vi "testTwoClientsSendCmdAtSameTime.vi"(8 "error in":errorcluster) -> (0 "error out":errorcluster)   [LabVIEW 2018]
uses:
  src/FactoryTcpServer/FactoryTcpServer.lvclass
  <vilib>/addons/_JKI Toolkits/Caraya/classes/Assert/Assert Equal Value_Variant.vi
  src/TcpServer/TcpServer.lvclass
  <vilib>/addons/_JKI Toolkits/Caraya/classes/Test/Test.lvclass
  <vilib>/addons/_JKI Toolkits/Caraya/classes/Assert/Assert.lvclass
panel:
  out "Run Server B error":errorcluster
  out "Run Server A error":errorcluster
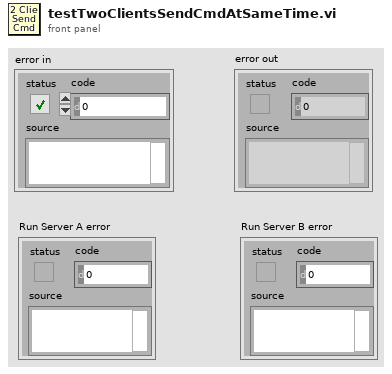
[diagram p1: front panel]
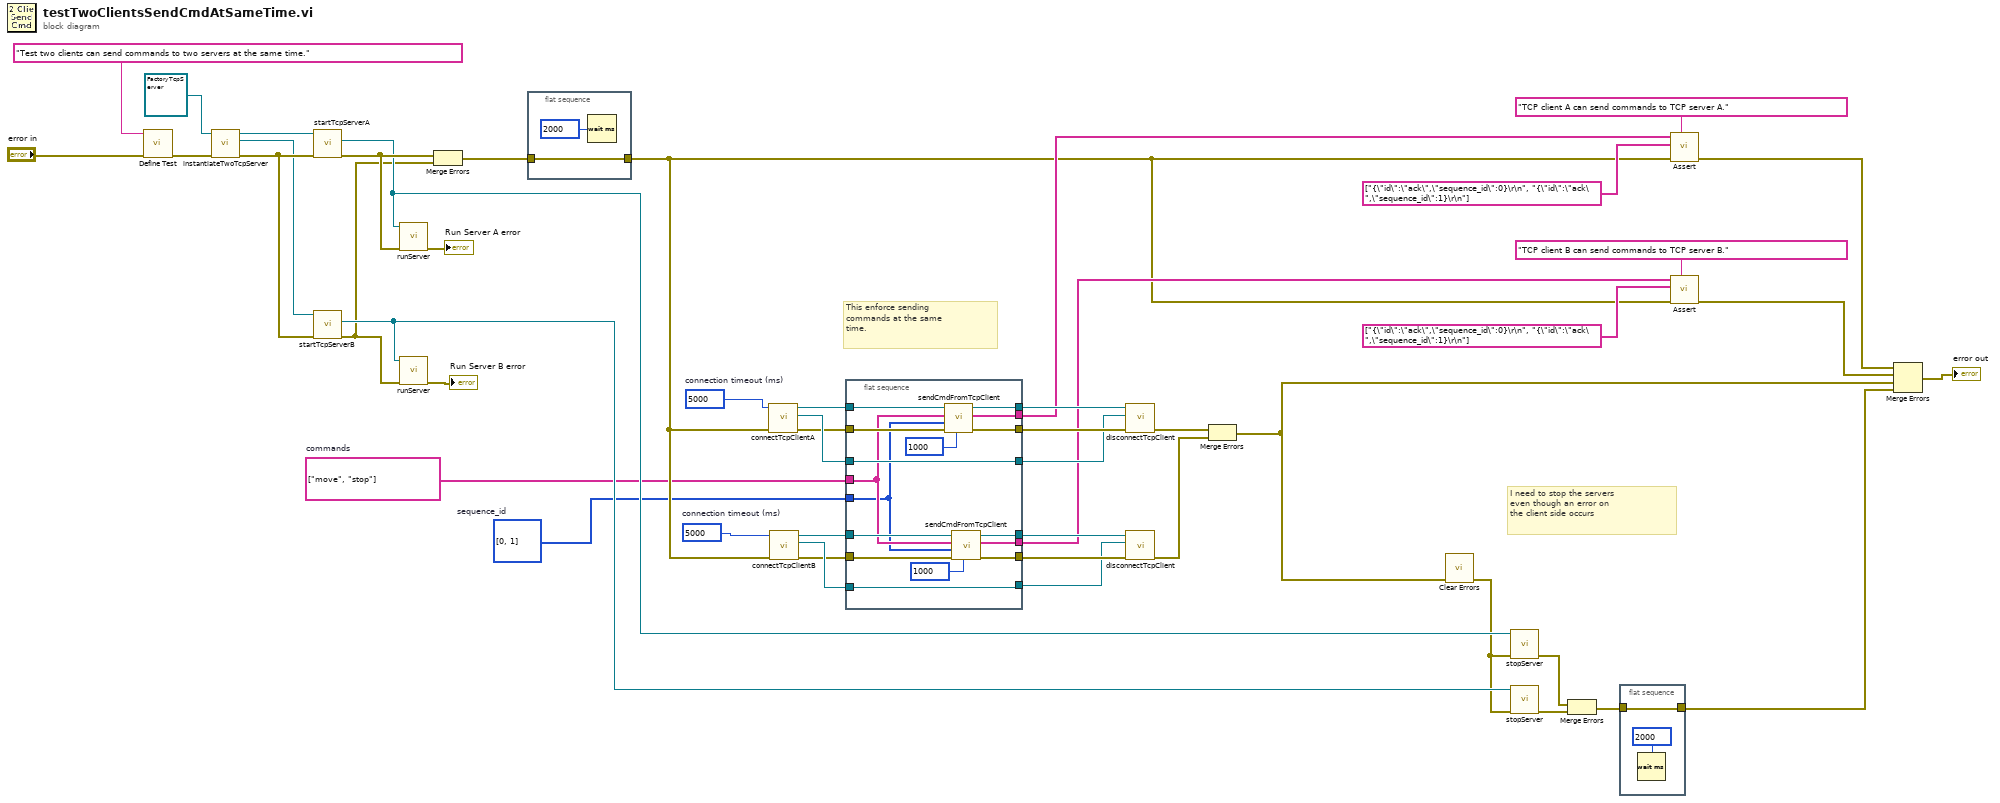
[diagram p0: block diagram]
diagram:
  w6 = 5000  # connection timeout (ms)
  w7 = 5000  # connection timeout (ms)
  w10 = i32[] [0, 1]  # sequence_id
  w11 = string[] ["move", "stop"]  # commands
  # "I need to stop the servers \neven though an error on \nthe client side occurs"
  # "This enforce sending\ncommands at the same\ntime."
  n1 = call <vilib>:"Define Test.vi"("error in (no error)"="error in", "Label (VI Title)"="Test two clients can send commands to two servers at the same time.") -> ("error out"=w5:errorcluster)  [unwired: 9 in]
  n2 = call "instantiateTwoTcpServer.vi"("error in (no error)"=w5, "FactoryTcpServer in"=refnum<class "FactoryTcpServer.lvclass"> refnum) -> ("error out"=w4:errorcluster, "TcpServer 2 out"=w2:refnum<class "TcpServer.lvclass">, "TcpServer 1 out"=w3:refnum<class "TcpServer.lvclass">)  [unwired: 6 in, 1 out]
  n3 = call "startTcpServerA.vi"("error in (no error)"=w4, "TcpServer.lvclass"=w3) -> ("error out"=w47:errorcluster, "TcpServer out"=w46:refnum<class "TcpServer.lvclass">)  [unwired: 7 in, 1 out]
  n4 = call "startTcpServerB.vi"("error in (no error)"=w4, "TcpServer.lvclass"=w2) -> ("error out"=w8:errorcluster, "TcpServer out"=w19:refnum<class "TcpServer.lvclass">)  [unwired: 7 in, 1 out]
  n5 = call "runServer.vi"("error in (no error)"=w47, "TcpServer in"=w46) -> ("error out (no error)"=→"Run Server A error":errorcluster)  [unwired: 8 in, 1 out]
  n6 = call "runServer.vi"("error in (no error)"=w8, "TcpServer in"=w19) -> ("error out (no error)"=→"Run Server B error":errorcluster)  [unwired: 8 in, 1 out]
  n7 = Merge Errors(w47, w8) -> (w9:errorcluster)
  n8 = flat-sequence {
    tunnel: w9 -> [w49]
    tunnel: [w49] -> w15
    frame #0 {
      n9 = Wait (ms)(milliseconds to wait=u32 2000) -> ()  [unwired: 1 out]
    }
  }
  n10 = call "connectTcpClientA.vi"("error in (no error)"=w15, "connection timeout (ms)"=w7) -> ("error out"=w33:errorcluster, "tel connection ID A out"=w39:refnum<k5>, "cmd connection ID A out"=w40:refnum<k5>)  [unwired: 7 in]
  n11 = call "connectTcpClientB.vi"("error in (no error)"=w15, "connection timeout (ms)"=w6) -> ("error out"=w26:errorcluster, "tel connection ID B out"=w27:refnum<k5>, "cmd connection ID B out"=w28:refnum<k5>)  [unwired: 7 in]
  n12 = flat-sequence {
    tunnel: [w64] -> w37
    tunnel: w40 -> [w65]
    tunnel: [w63] -> w36
    tunnel: [w66] -> w35
    tunnel: w39 -> [w66]
    tunnel: w33 -> [w62]
    tunnel: [w61] -> w31
    tunnel: w28 -> [w60]
    tunnel: [w59] -> w23
    tunnel: w27 -> [w59]
    tunnel: w26 -> [w58]
    tunnel: [w57] -> w25
    tunnel: [w56] -> w24
    tunnel: [w55] -> w20
    tunnel: w11 -> [w54]
    tunnel: w10 -> [w53]
    frame #0 {
      n13 = call "sendCmdFromTcpClient.vi"("timeout ms (1000)"=1000, "error in (no error)"=w62, "sequence_id"=w53, "commands"=w54, "connectionID"=w65) -> ("error out"=w63:errorcluster, "ack received"=w61:string[], "connectionID"=w64:refnum<k5>)  [unwired: 4 in]
      n14 = call "sendCmdFromTcpClient.vi"("timeout ms (1000)"=1000, "error in (no error)"=w58, "sequence_id"=w53, "commands"=w54, "connectionID"=w60) -> ("error out"=w56:errorcluster, "ack received"=w55:string[], "connectionID"=w57:refnum<k5>)  [unwired: 4 in]
    }
  }
  n15 = call "disconnectTcpClient.vi"("error in (no error)"=w36, "tel connection ID in"=w35, "cmd connection ID in"=w37) -> ("error out"=w34:errorcluster)  [unwired: 8 in]
  n16 = call "disconnectTcpClient.vi"("error in (no error)"=w24, "tel connection ID in"=w23, "cmd connection ID in"=w25) -> ("error out"=w16:errorcluster)  [unwired: 8 in]
  n17 = Merge Errors(w34, w16) -> (w13:errorcluster)
  n18 = call <vilib>:"Clear Errors.vi"("error in (no error)"=w13) -> ("error out"=w12:errorcluster)  [unwired: 5 in, 1 out]
  n19 = call "stopServer.vi"("error in (no error)"=w12, "tcpServer in"=w46) -> ("error out"=w43:errorcluster)  [unwired: 8 in, 1 out]
  n20 = call "stopServer.vi"("error in (no error)"=w12, "tcpServer in"=w19) -> ("error out"=w42:errorcluster)  [unwired: 8 in, 1 out]
  n21 = Merge Errors(w43, w42) -> (w41:errorcluster)
  n22 = flat-sequence {
    tunnel: w41 -> [w67]
    tunnel: [w67] -> w14
    frame #0 {
      n23 = Wait (ms)(milliseconds to wait=u32 2000) -> ()  [unwired: 1 out]
    }
  }
  n24 = call-poly <vilib>:"Assert.vi"("Label"="TCP client A can send commands to TCP server A.", "error in (no error)"=w15, "Y"=string[] ["{\"id\":\"ack\",\"sequence_id\":0}\r\n", "{\"id\":\"ack\",\"sequence_id\":1}\r\n"] ("ack received"), "X"=w31) -> ("error out"=w18:errorcluster)  [unwired: 7 in]
  n25 = call-poly <vilib>:"Assert.vi"("Label"="TCP client B can send commands to TCP server B.", "error in (no error)"=w15, "Y"=string[] ["{\"id\":\"ack\",\"sequence_id\":0}\r\n", "{\"id\":\"ack\",\"sequence_id\":1}\r\n"] ("ack received"), "X"=w20) -> ("error out"=w17:errorcluster)  [unwired: 7 in]
  n26 = Merge Errors(w18, w17, w13, w14) -> (→"error out":errorcluster)
